vi "Actor.vi"(4 "Queue of Error":refnum<queue>, 6 "Queue of Self Attributes":refnum<queue>, 9 "Refs":refnum<class "Refs.lvclass">, 10 "Attributes":refnum<class "Attributes.lvclass">, 11 "TEMPLATE Actor in":refnum<class "TEMPLATE Actor.lvclass">) -> (0 "Error out":errorcluster, 3 "TEMPLATE Actor out":refnum<class "TEMPLATE Actor.lvclass">)   [LabVIEW 2025, in "_Template.lvlib" / "Templates.lvlib" / "TEMPLATE Actor.lvlib" / "TEMPLATE Actor.lvclass"]
uses:
  TEMPLATE Actor.lvclass
  C:/git/jettl/src/jettl/jettl/Actor/Actor.lvclass
  jettl/jettl/Refs/Refs.lvclass
  jettl/jettl/Attributes/Attributes/Attributes.lvclass
  Refs.ctl
  TEMPLATE Actor.lvlib
  jettl/jettl/jettl.lvlib
  jettl/jettl/Transport/Event/Event.lvlib
types:
  T1 = typedef "_Template.lvlib/Templates.lvlib/TEMPLATE Actor.lvlib/Refs.ctl" = cluster{"placeholder":refnum<vi>}
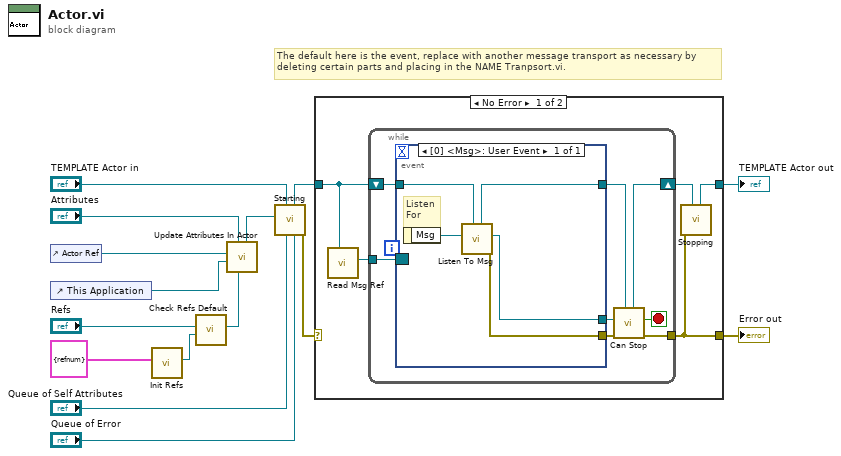
[diagram p0: block diagram]
diagram:
  # "The default here is the event, replace with another message transport as necessary by deleting certain parts and placing in the NAME Tranpsort.vi."
  n1 = control-ref of="Actor Ref"() -> (w9:refnum<vi>)
  n2 = control-ref of="This Application"() -> (w8:refnum<vi>)
  n3 = call "Init Refs.vi"("Refs"=T1 {"placeholder"=refnum} ("Control Refs")) -> ("Refs"=w10:refnum<class "Refs.lvclass">)  [unwired: 10 in]
  n4 = call "Check Refs Default.vi"("Refs (Instantiated In Actor)"=w10, "Refs"="Refs") -> ("Refs"=w7:refnum<class "Refs.lvclass">)  [unwired: 9 in]
  n5 = call "Update Attributes In Actor.vi"("Refs"=w7, "Attributes in"="Attributes", "Application Ref"=w8, "Actor Ref"=w9) -> ("Attributes out"=w4:refnum<class "Attributes.lvclass">)  [unwired: 7 in]
  n6 = call "Starting.vi"("Queue of Error"="Queue of Error", "Queue of Self Attributes"="Queue of Self Attributes", "Actor in"="TEMPLATE Actor in", "Attributes"=w4) -> ("Error out"=w3:errorcluster, "Actor out"=w5:refnum<class "TEMPLATE Actor.lvclass">)  [unwired: 6 in]
  n7 = case shown="No Error" w3 {
    selector: w3 -> [_ w34]
    tunnel: [w18 w35] -> w14
    tunnel: w5 -> [w17 w35]
    tunnel: [w20 w34] -> w15
    frame No Error {
      n8 = call "Read Msg Ref.vi"("Actor"=w17) -> ("Msg Ref"=w16:refnum<event-registration>)  [unwired: 10 in]
      n9 = while {
        shift-right: [w24] -> w19
        shift-left: w17 -> [w27]
        tunnel: w16 -> [w28]
        tunnel: [w25] -> w20
        stop <- w23 stop-if-true
        n10 = event shown="[0] <Msg>: User Event" {
          selector: w28 -> [_]
          dyn-events: _ -> [_]
          timeout: _ -> [_]
          tunnel: w27 -> [w33]
          tunnel: [w31] -> w22
          tunnel: [w30] -> w26
          tunnel: [w29] -> w21
          event User Event {
            # "Listen\nFor"
            n11 = event-data() -> ("Msg"=w32:refnum<class "Msg.lvclass">)  [unwired: 1 in]
            n12 = call "Listen To Msg.vi"("Actor in"=w33, "Msg"=w32) -> ("Error out"=w30:errorcluster, "Msg Output"=w29:refnum<class "Msg Output.lvclass">, "Actor out"=w31:refnum<class "TEMPLATE Actor.lvclass">)  [unwired: 7 in]
          }
        }
        n13 = call "Can Stop.vi"("Actor in"=w22, "Error in"=w26, "Msg Output"=w21) -> ("Error out"=w25:errorcluster, "Stop"=w23:bool, "Actor out"=w24:refnum<class "TEMPLATE Actor.lvclass">)  [unwired: 6 in]
      }
      n14 = call "Stopping.vi"("Actor in"=w19, "Error in"=w20) -> ("Actor out"=w18:refnum<class "TEMPLATE Actor.lvclass">)  [unwired: 9 in]
    }
    frame Error {
    }
  }
  "TEMPLATE Actor out" <- w14
  "Error out" <- w15
